vi "SCP Open.vi"(8 "Error In":errorcluster, 9 "Password":string, 10 "Username":string, 11 "Hostname or IP":string) -> (0 "Error Out":errorcluster, 2 "Connected?":bool, 3 "SCP Session":refnum<k24>)   [LabVIEW 2014, in "LMH-LINX.lvlib"]
uses:
  <vilib>/MakerHub/LINX/LMH-LINX.lvlib
  C:/Program Files (x86)/National Instruments/LabVIEW 2014/vi.lib/MakerHub/LINX/Resources/Renci.SshNet.dll
  Resources/Renci.SshNet.dll
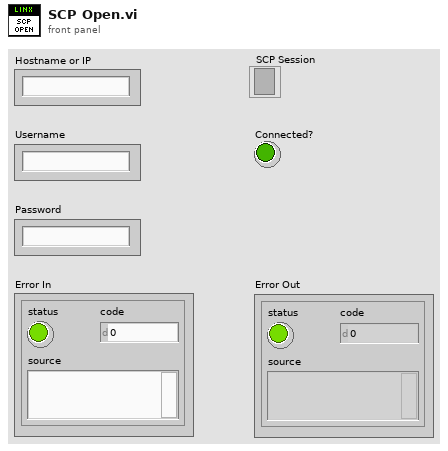
[diagram p1: front panel]
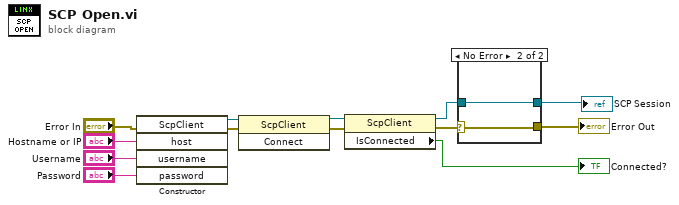
[diagram p0: block diagram]
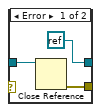
[diagram p2: hidden frame]
diagram:
  n1 = constructor class="ScpClient"(error in="Error In", "host"="Hostname or IP", "username"="Username", "password"="Password") -> (reference out=w7:refnum<k24>, error out=w8:errorcluster)  [unwired: 2 in, 4 out]
  n2 = invoke class="ScpClient" method="Connect"(reference=w7, error in=w8) -> (reference out=w6:refnum<k24>, error out=w5:errorcluster)  [unwired: 1 in, 1 out]
  n3 = property class="ScpClient"(reference=w6, error in=w5) -> (reference out=w2:refnum<k24>, error out=w4:errorcluster, "IsConnected"=→"Connected?":bool)
  n4 = case shown="No Error" w4 {
    selector: w4 -> [_ w18]
    tunnel: [w15 w18] -> w3
    tunnel: [refnum<k0> refnum w17] -> w1
    tunnel: w2 -> [w14 w17]
    frame Error {
      n5 = Close Reference(reference=w14) -> (error out=w15:errorcluster)  [unwired: 1 in]
    }
    frame No Error {
    }
  }
  "Error Out" <- w3
  "SCP Session" <- w1
